vi "RSZVB Get Same Sweep Setup.vi"(8 "error in (no error)":errorcluster {"code" format="%.0x"}, 9 "Channel (1)":i32=1, 11 "VISA session":refnum<visa-resource-name>) -> (0 "error out":errorcluster {"code" format="%.0x"}, 2 "Same Sweep Setup":bool, 3 "dup VISA session":refnum<visa-resource-name>)   [LabVIEW 2011]
doc: "This VI returns the sweep setup for the calibration sweeps.\n\nRemote-control command(s):\n[SENSe<Ch>:]CORRection:COLLect:CSETup?"
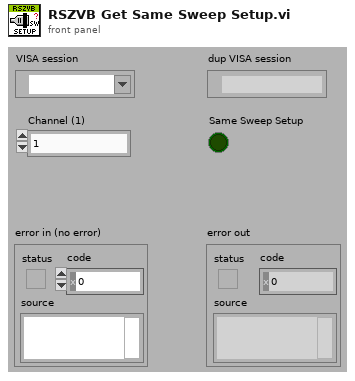
[diagram p1: front panel]
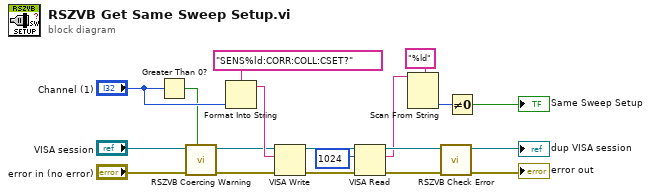
[diagram p0: block diagram]
diagram:
  n1 = Greater Than 0?(x="Channel (1)") -> (x > 0?=w1:bool)
  n2 = call "RSZVB Coercing Warning.vi"("In Range?"=w1, "error in (no error)"="error in (no error)", "VISA session"="VISA session") -> ("error out"=w16:errorcluster, "dup VISA session"=w18:refnum<visa-resource-name>)  [unwired: 7 in]
  n3 = Format Into String(format string="SENS%ld:CORR:COLL:CSET?", "Channel (1)") -> (resulting string=w19:string)  [unwired: 2 in, 1 out]
  n4 = VISA Write(VISA resource name=w18, write buffer=w19, error in (no error)=w16) -> (VISA resource name out=w13:refnum<visa-resource-name>, error out=w12:errorcluster)  [unwired: 1 out]
  n5 = VISA Read(VISA resource name=w13, byte count=u32 1024 ("byte count (0)"), error in (no error)=w12) -> (VISA resource name out=w11:refnum<visa-resource-name>, read buffer=w8:string, error out=w15:errorcluster)  [unwired: 1 out]
  n6 = Scan From String(format string="%ld", input string=w8) -> (output 1=w9:i32)  [unwired: 3 in, 3 out]
  n7 = call "RSZVB Check Error.vi"("error in (no error)"=w15, "VISA session"=w11) -> ("error out"=→"error out":errorcluster, "dup VISA session"=→"dup VISA session":refnum<visa-resource-name>)  [unwired: 8 in]
  n8 = Not Equal To 0?(x=w9) -> (x != 0?=→"Same Sweep Setup":bool)
